vi "frequencies_from_range_parameters.vi"(7 "Center frequency (Hz)":dbl=32768.0, 8 "Fine increment (Hz)":dbl=0.5, 9 "Fine range width (Hz)":dbl=5.0, 10 "Coarse increment (Hz)":dbl=1.0, 11 "Coarse range width (Hz)":dbl=40.0) -> (0 "Fine range end (Hz)":dbl=32773.0, 1 "Fine range start (Hz)":dbl=32763.0, 2 "Coarse range end (Hz)":dbl=32813.0, 3 "Coarse range start (Hz)":dbl=32723.0, 5 "Measurement frequencies (Hz)":dbl[](array[numeric])=[32723.0, 32724.0, 32725.0, 32726.0, 32727.0, 32728.0, 32729.0, 32730.0, 32731.0, 32732.0, 32733.0, 32734.0, 32735.0, 32736.0, 32737.0, 32738.0, 32739.0, 32740.0, 32741.0, 32742.0, 32743.0, 32744.0, 32745.0, 32746.0, 32747.0, 32748.0, 32749.0, 32750.0, 32751.0, 32752.0, 32753.0, 32754.0, 32755.0, 32756.0, 32757.0, 32758.0, 32759.0, 32760.0, 32761.0, 32762.0, 32763.0, 32763.5, 32764.0, 32764.5, 32765.0, 32765.5, 32766.0, 32766.5, 32767.0, 32767.5, 32768.0, 32768.5, 32769.0, 32769.5, 32770.0, 32770.5, 32771.0, 32771.5, 32772.0, 32772.5, 32773.0, 32774.0, 32775.0, 32776.0, 32777.0, 32778.0, 32779.0, 32780.0, 32781.0, 32782.0, 32783.0, 32784.0, 32785.0, 32786.0, 32787.0, 32788.0, 32789.0, 32790.0, 32791.0, 32792.0, 32793.0, 32794.0, 32795.0, 32796.0, 32797.0, 32798.0, 32799.0, 32800.0, 32801.0, 32802.0, 32803.0, 32804.0, 32805.0, 32806.0, 32807.0, 32808.0, 32809.0, 32810.0, 32811.0, 32812.0, 32813.0])   [LabVIEW 2020, in "Resonance Curve Data.lvclass"]
uses:
  Resonance Curve Data.lvclass
  Resonance Curve Data.lvclass/Resonance Curve Data.ctl
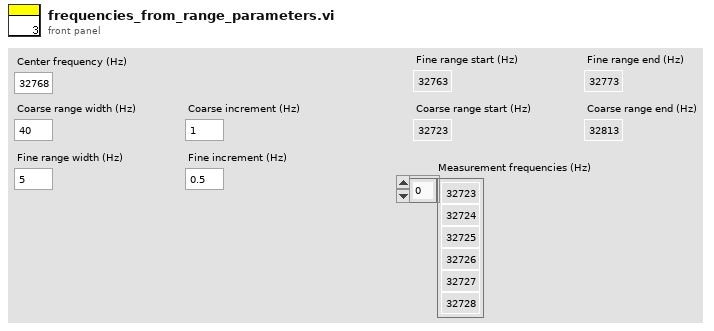
[diagram p1: front panel]
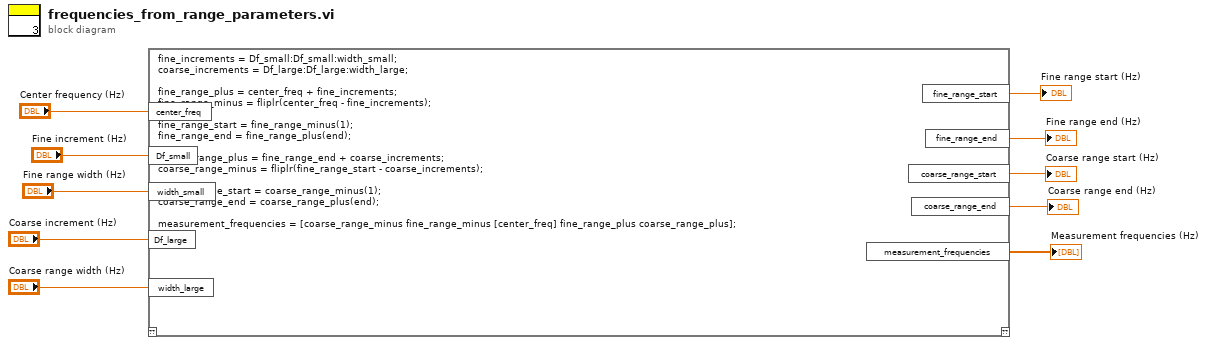
[diagram p0: block diagram]
diagram:
  n1 = script code="fine_increments = Df_small:Df_small:width_small;\ncoarse_increments = Df_large:Df_large:width_large;\n\nfine_range_plus = center_freq + fine_increments;\nfine_range_minus = fliplr(center_freq - fine_increments);\n\nfine_range_start = fine_range_minus(1);\nfine_range_end = fine_range_plus(end);\n\ncoarse_range_plus = fine_range_end + coarse_increments;\ncoarse_range_minus = fliplr(fine_range_start - coarse_increments);\n\ncoarse_range_start = coarse_range_minus(1);\ncoarse_range_end = coarse_range_plus(end);\n\nmeasurement_frequencies = [coarse_range_minus fine_range_minus [center_freq] fine_range_plus coarse_range_plus];"("center_freq"="Center frequency (Hz)", "Df_small"="Fine increment (Hz)", "width_small"="Fine range width (Hz)", "Df_large"="Coarse increment (Hz)", "width_large"="Coarse range width (Hz)") -> ("fine_range_start"=→"Fine range start (Hz)":dbl, "fine_range_end"=→"Fine range end (Hz)":dbl, "coarse_range_start"=→"Coarse range start (Hz)":dbl, "coarse_range_end"=→"Coarse range end (Hz)":dbl, "measurement_frequencies"=→"Measurement frequencies (Hz)":dbl[])  [unwired: 1 in, 1 out]
